vi "Importer.vi"() -> ()   [LabVIEW 2013]
uses:
  Database/Database.lvclass
  <vilib>/addons/database/_DB Variant To Data/Database Variant To Data.xnode
panel:
  in  "mouse tuple":T1={"mouse_id"=1217.0, "mouse_gender"="male", "mouse_strain"="C57BL6/J", "mouse_dob"="", "mouse_dod"="", "mouse_notes"="", "headpost_date"=""}
  out "error":bool
  in  "Import":bool
  in  "stop":bool
  in  "Exo Tuple":T2={"mouse_id"=1217.0, "exp_date"="", "operator"="Manolis", "mass"=0.0, "anesthesia"="fentanyl", "directory"="", "dyes"="OGB", "exp_notes"="", "setup"="2P1", "archive"="", "process"="yes"}
  in  "Tab Control":enum32{"Mouse/Experiment", "Scans"}(tab)
  in  "Archive":string="2PS1A4"
  in  "dyes":string(combo)="OGB"
  in  "Directory":string
  in  "Anesthesia":string(combo)="fentanyl"
  in  "Weight":dbl
  in  "Gender":string(combo)="male"
  in  "Strain":string(combo)="C57BL6/J"
  in  "Birthday":string
  in  "ID":dbl
  in  "Session":path=path "Z:/users/Manolis/Labview/Scanner/sessions_Win7.dsn"
  in  "Mag":dbl=1.0
  in  "Rot":dbl
  in  "Aim":string(combo)="vesselMap"
  in  "Idx":dbl=1.0
  in  "cell #":dbl
  in  "Notes":string
  in  "State":string(combo)="anesthetized"
  in  "File Name":string="vessels"
  in  "Scan Prog":string(combo)="Imager"
  in  "Surface":dbl
  in  "Stim":string(combo)="None"
  in  "Scans":string[][](table)
  in  "Tuple":T3={"mouse_id"=1217.0, "exp_date"="2013-05-16", "scan_idx"=33.0, "file_name"="test", "scan_prog"="Imager", "aim"="other", "stim_engine"="None", "Lens"=0.0, "mag"=0.0, "laser_wavelength"=0.0, "attenuator_setting"=0.0, "x"=0.0, "y"=0.0, "z"=0.0, "surfz"=0.0, "scan_rotation"=0.0, "notes"="", "cell_patch"=0.0, "state"="", "problem_type"=""}
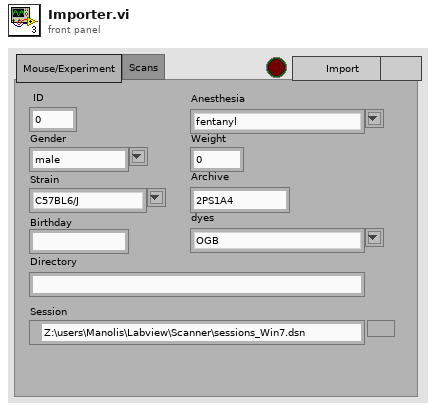
[diagram p1: front panel]
types:
  T1 = cluster{"mouse_id":dbl, "mouse_gender":string, "mouse_strain":string, "mouse_dob":string, "mouse_dod":string, "mouse_notes":string, "headpost_date":string}
  T2 = cluster{"mouse_id":dbl, "exp_date":string, "operator":string, "mass":dbl, "anesthesia":string, "directory":string, "dyes":string, "exp_notes":string, "setup":string, "archive":string, "process":string}
  T3 = cluster{"mouse_id":dbl, "exp_date":string, "scan_idx":dbl, "file_name":string, "scan_prog":string, "aim":string, "stim_engine":string, "Lens":dbl, "mag":dbl, "laser_wavelength":dbl, "attenuator_setting":dbl, "x":dbl, "y":dbl, "z":dbl, "surfz":dbl, "scan_rotation":dbl, "notes":string, "cell_patch":dbl, "state":string, "problem_type":string}
  T4 = cluster{"scan_idx":string, "lens":string, "mag":string, "x":string, "y":string, "z":string, "scan_rotation":string, "scan_prog":string}[]
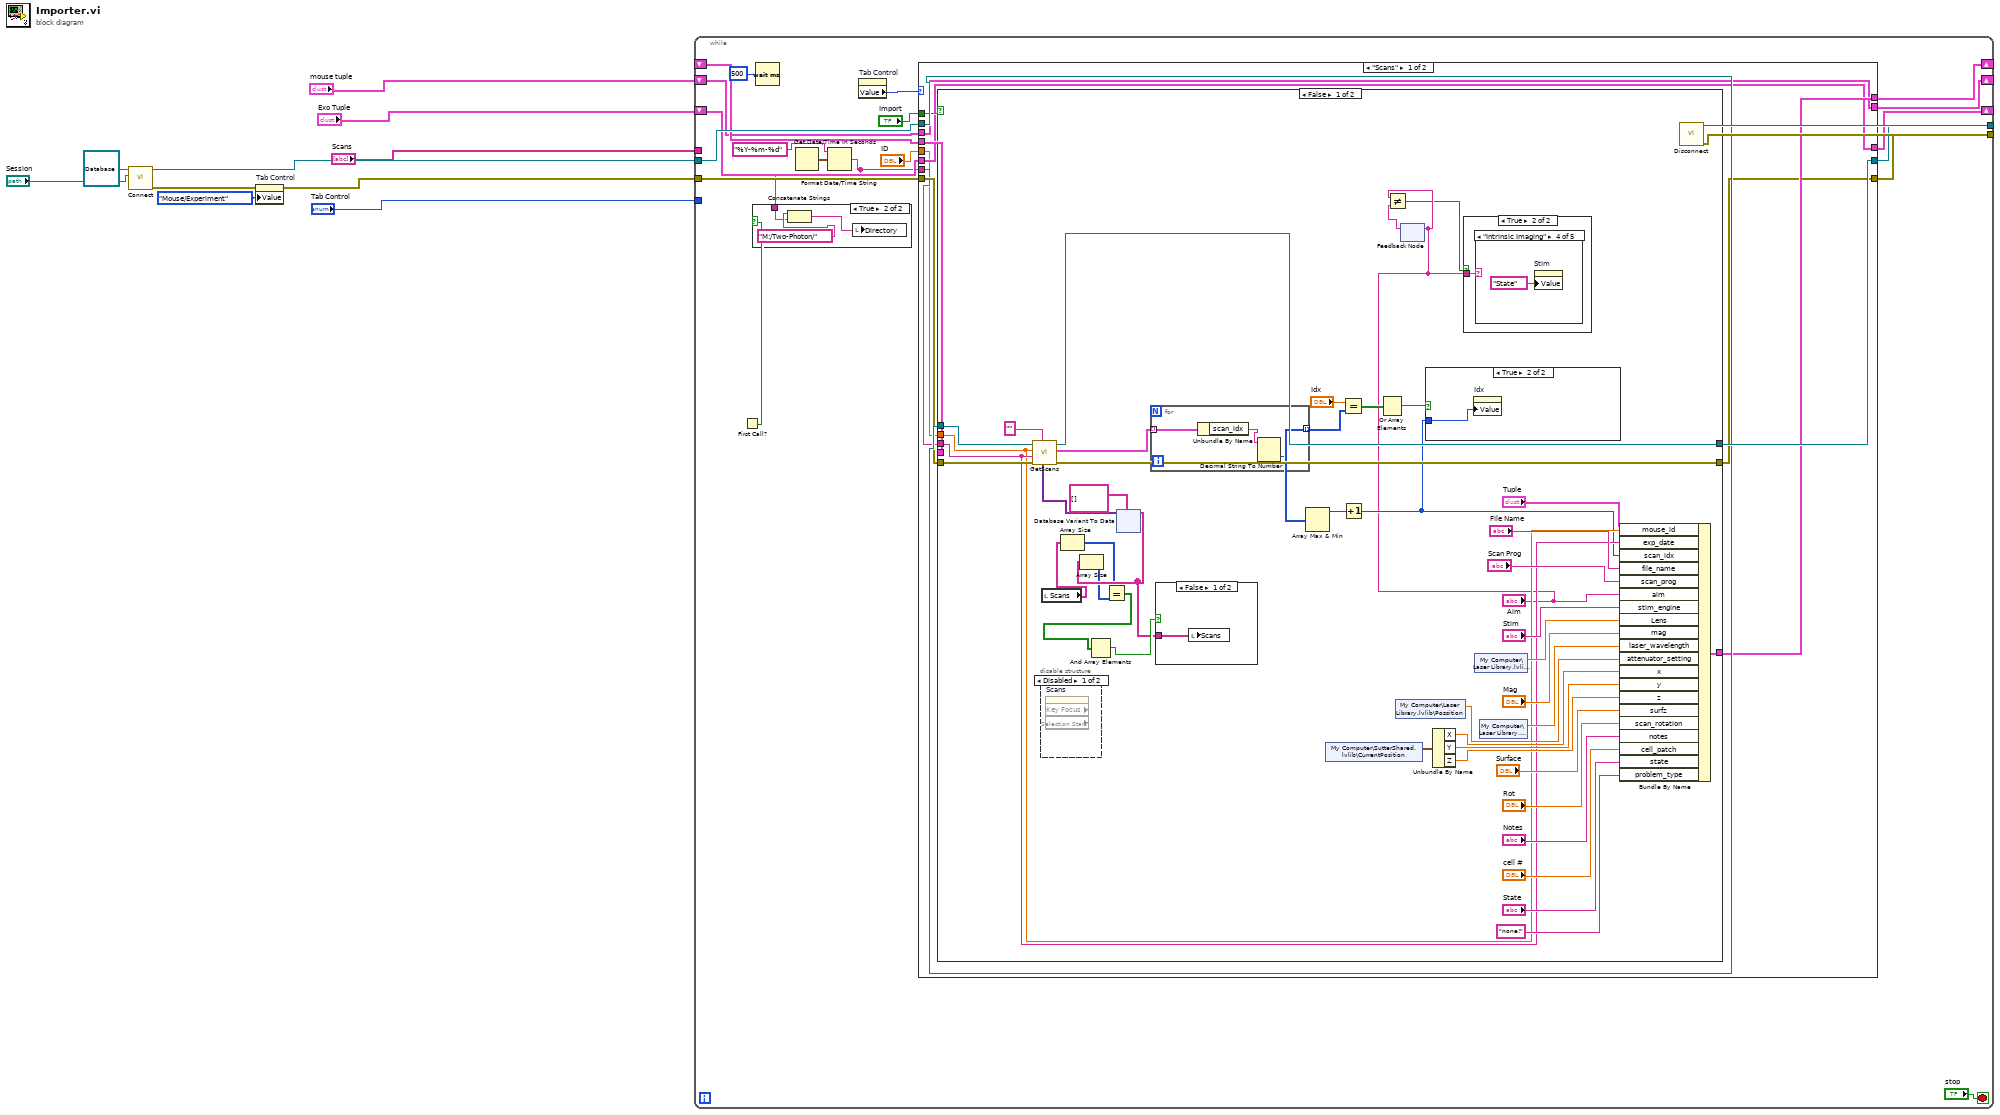
[diagram p0: block diagram]
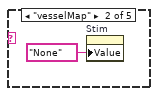
[diagram p5: hidden frame]
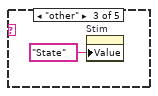
[diagram p6: hidden frame]
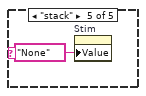
[diagram p7: hidden frame]
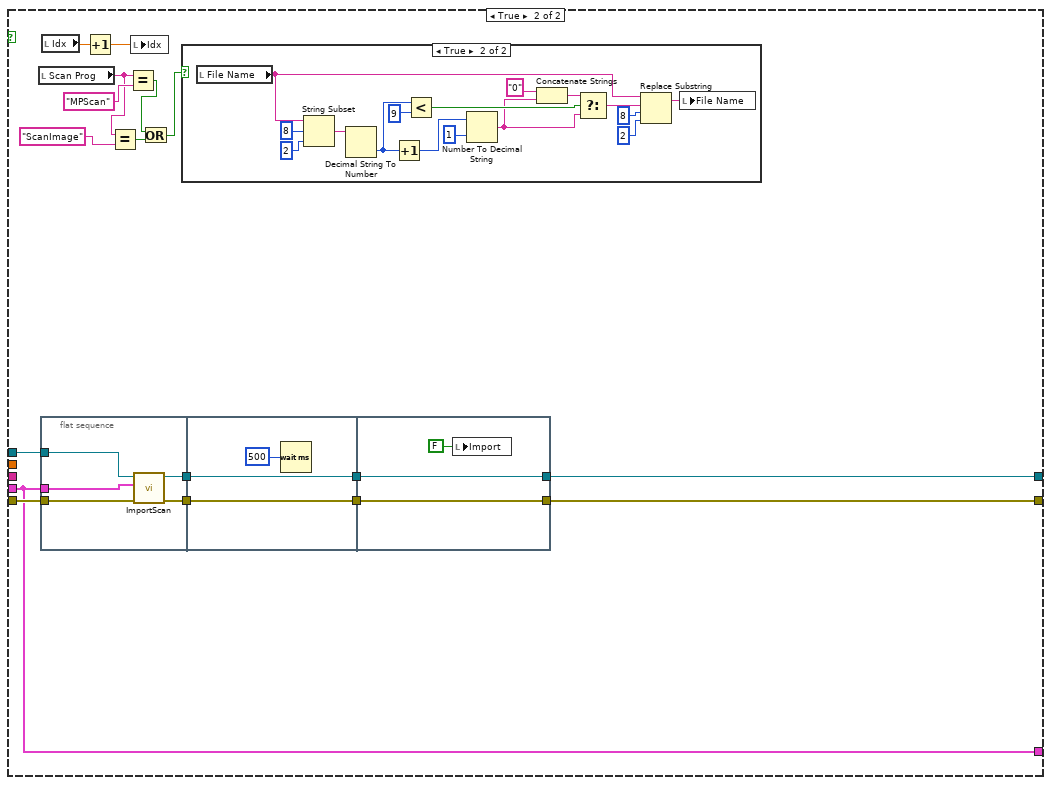
[diagram p11: hidden frame]
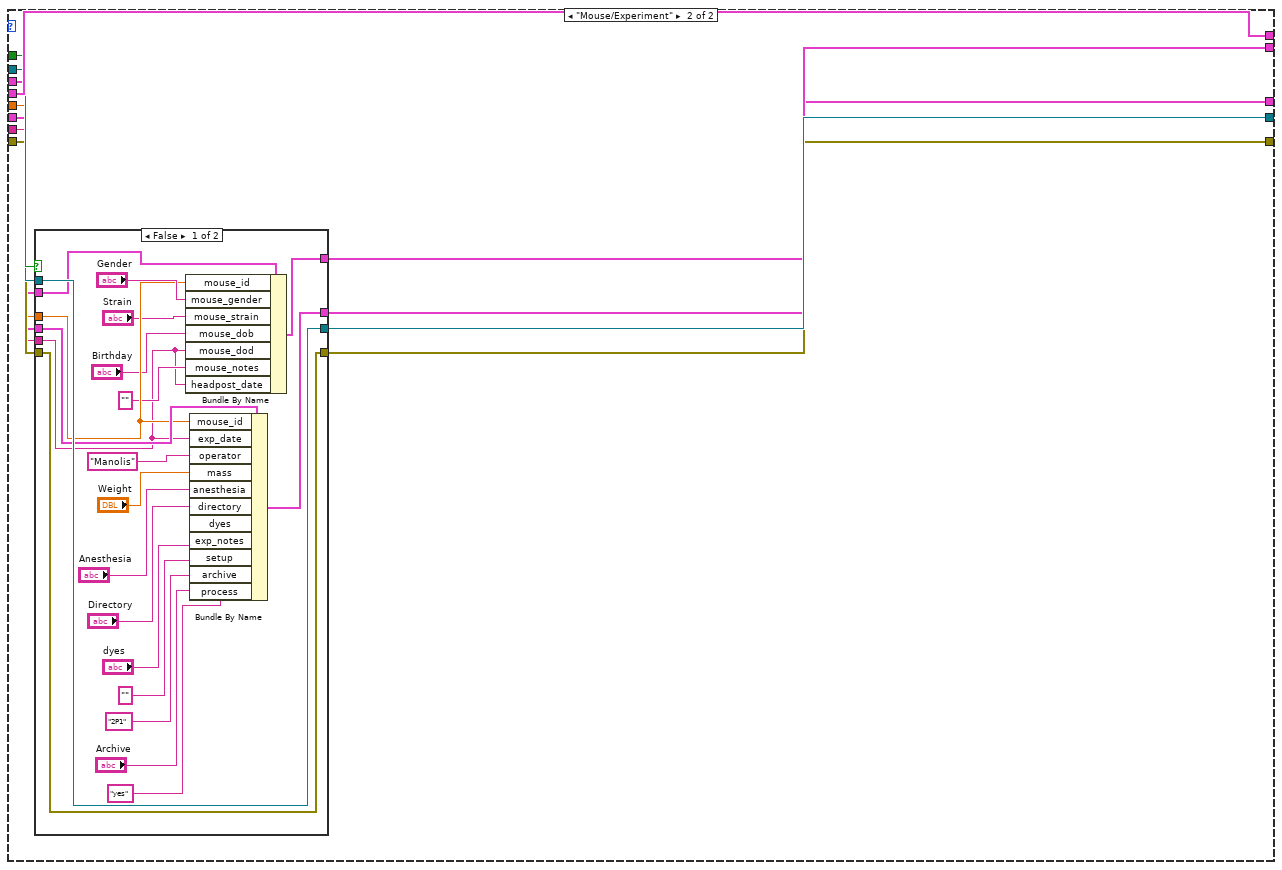
[diagram p13: hidden frame]
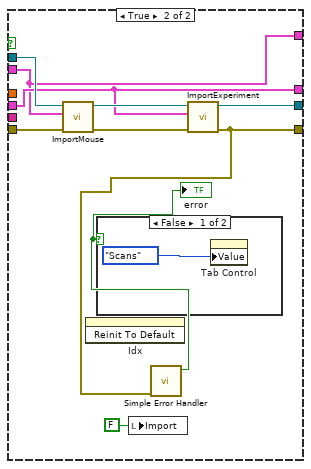
[diagram p14: hidden frame]
diagram:
  n1 = call-dynamic "Connect.vi"("Session"="Session", "Database in"=refnum<class "Database.lvclass"> refnum) -> ("error out"=w4:errorcluster, "Database out"=w10:refnum<class "Database.lvclass">)  [unwired: 8 in]
  n2 = property on="Tab Control" class="TabCtl (strict)"(error in=w4, "Value"=enum32{"Mouse/Experiment", "Scans"}."Mouse/Experiment" ("Tab Control")) -> (error out=w3:errorcluster)  [unwired: 1 in, 1 out]
  n3 = while {
    tunnel: [w31] -> w11
    tunnel: w10 -> [w30]
    tunnel: w3 -> [w28]
    tunnel: [w25] -> w8
    shift-right: [w26] -> _
    shift-left: _ -> [w27]
    tunnel: "Scans" -> [_]
    tunnel: "Tab Control" -> [_]
    shift-right: [w20] -> _
    shift-left: "mouse tuple" -> [w21]
    shift-right: [w18] -> _
    shift-left: "Exo Tuple" -> [w19]
    stop <- "stop" stop-if-true
    n4 = First Call?() -> (First Call?: T/F=w14:bool)
    n5 = Wait (ms)(milliseconds to wait=u32 500) -> ()  [unwired: 1 out]
    n6 = Get Date/Time In Seconds() -> (seconds since 1Jan1904=w23:timestamp)
    n7 = Format Date/Time String(time format string (%c)="%Y-%m-%d", seconds (now)=w23) -> (date/time string=w13:string)  [unwired: 1 in]
    n8 = case shown="True" w14 {
      tunnel: w13 -> [_ w32]
      frame False {
      }
      frame True {
        n9 = Concatenate Strings("M:/Two-Photon/" ("Directory"), w32) -> (w33:string)
        n10 = local write "Directory"(w33) -> ()
      }
    }
    n11 = property on="Tab Control" class="TabCtl (strict)"() -> ("Value"=w16:enum32{"Mouse/Experiment", "Scans"})  [unwired: 2 in, 2 out]
    n12 = case shown="\"Scans\"" w16 {
      tunnel: [w45 w196] -> w31
      tunnel: w30 -> [w44 w197]
      tunnel: w28 -> [w43 w194]
      tunnel: w27 -> [w42 w199]
      tunnel: [w41 w199] -> w26
      tunnel: [w40 w195] -> w25
      tunnel: w13 -> [w39 w188]
      tunnel: "Import" -> [w38 w198]
      tunnel: w21 -> [w37 w193]
      tunnel: [w37 w192] -> w20
      tunnel: w19 -> [w36 w191]
      tunnel: [w36 w190] -> w18
      tunnel: "ID" -> [w35 w189]
      frame "Scans" {
        n13 = case shown="False" w38 {
          tunnel: [w69 w160] -> w45
          tunnel: w44 -> [w70 w159]
          tunnel: w43 -> [w67 w158]
          tunnel: [w66 w157] -> w40
          tunnel: w42 -> [_ w156]
          tunnel: [w72 w156] -> w41
          tunnel: w39 -> [w65 _]
          tunnel: w35 -> [w64 _]
          frame False {
            n14 = call-dynamic "GetScans.vi"("condition"="", "error in (no error)"=w67, "exp_date"=w65, "mouse_id"=w64, "Database in"=w70) -> ("error out"=w66:errorcluster, "Scan Clusters"=w62:T4, "Database out"=w69:refnum<class "Database.lvclass">, "data"=w63:variant[][])  [unwired: 2 in]
            n15 = disable-structure shown="Disabled" {
              frame Disabled {
                n16 = property on="Scans" class="Tbl (strict)" props=["Key Focus", "Selection Start"]() -> ()  [unwired: 2 in, 4 out]
              }
              frame Enabled {
              }
            }
            n17 = local read "Scans"() -> (w51:string[][])
            n18 = Array Size(array=w51) -> (size(s)=w49:i32[])
            n19 = xnode "Database Variant To Data"("database variant"=w63, "type"=string[][] []) -> ("data"=w52:string[][])  [unwired: 1 in, 1 out]
            n20 = Array Size(array=w52) -> (size(s)=w50:i32[])
            n21 = Equal?(x=w49, y=w50) -> (x = y?=w53:bool[])
            n22 = And Array Elements(Boolean array=w53) -> (logical AND=w54:bool)
            n23 = for {
              tunnel: w62 -> [w99] mode=indexing
              tunnel: [w97] -> w60 mode=indexing
              n24 = Unbundle By Name(w99) -> ("scan_idx"=w98:string)
              n25 = Decimal String To Number(string=w98) -> (number=w97:i32)  [unwired: 2 in, 1 out]
            }
            n26 = case shown="False" w54 {
              tunnel: w52 -> [w95 _]
              frame False {
                n27 = local write "Scans"(w95) -> ()
              }
              frame True {
              }
            }
            n28 = Array Max & Min(array=w60) -> (max value=w61:i32)  [unwired: 3 out]
            n29 = shared-variable "My Computer\\SutterShared.lvlib\\CurrentPosition"() -> (w89:cluster{"X":dbl, "Y":dbl, "Z":dbl, "Depth":dbl})  [unwired: 1 in, 1 out]
            n30 = Equal?(x="Idx", y=w60) -> (x = y?=w58:bool[])
            n31 = Increment(x=w61) -> (x+1=w56:i32)
            n32 = Or Array Elements(Boolean array=w58) -> (logical OR=w57:bool)
            n33 = shared-variable "My Computer\\Laser Library.lvlib\\Possition"() -> (w78:dbl)  [unwired: 1 in, 1 out]
            n34 = feedback-in #1("Aim") -> ()
            n35 = feedback #1() -> (w48:string)  [unwired: 1 in]
            n36 = Not Equal?(x="Aim", y=w48) -> (x != y?=w46:bool)
            n37 = case shown="True" w57 {
              tunnel: w56 -> [_ w96]
              frame False {
              }
              frame True {
                n38 = property on="Idx" class="DigNum (strict)"("Value"=w96) -> ()  [unwired: 2 in, 2 out]
              }
            }
            n39 = Unbundle By Name(w89) -> ("X"=w81:dbl, "Y"=w80:dbl, "Z"=w79:dbl)
            n40 = case shown="True" w46 {
              tunnel: "Aim" -> [_ w90]
              frame False {
              }
              frame True {
                n41 = case shown="\"Intrinsic Imaging\"" w90 {
                  frame "False", Default {
                  }
                  frame "vesselMap" {
                    n42 = property on="Stim" class="CmbBox"("Value"="None" ("Stim")) -> ()  [unwired: 2 in, 2 out]
                  }
                  frame "other" {
                    n43 = property on="Stim" class="CmbBox"("Value"="State" ("Stim")) -> ()  [unwired: 2 in, 2 out]
                  }
                  frame "Intrinsic Imaging" {
                    n44 = property on="Stim" class="CmbBox"("Value"="State" ("Stim")) -> ()  [unwired: 2 in, 2 out]
                  }
                  frame "stack" {
                    n45 = property on="Stim" class="CmbBox"("Value"="None" ("Stim")) -> ()  [unwired: 2 in, 2 out]
                  }
                }
              }
            }
            n46 = shared-variable "My Computer\\Laser Library.lvlib\\Lens"() -> (w76:dbl)  [unwired: 1 in, 1 out]
            n47 = shared-variable "My Computer\\Laser Library.lvlib\\WV"() -> (w77:dbl)  [unwired: 1 in, 1 out]
            n48 = Bundle By Name(cluster="Tuple", "mouse_id"=w64, "exp_date"=w65, "scan_idx"=w56, "file_name"="File Name", "scan_prog"="Scan Prog", "aim"="Aim", "stim_engine"="Stim", "Lens"=w76, "mag"="Mag", "laser_wavelength"=w77, "attenuator_setting"=w78, "x"=w81, "y"=w80, "z"=w79, "surfz"="Surface", "scan_rotation"="Rot", "notes"="Notes", "cell_patch"="cell #", "state"="State", "problem_type"="none!") -> (w72:T3)
          }
          frame True {
            n49 = local read "Scan Prog"() -> (w145:string)
            n50 = flat-sequence {
              tunnel: w159 -> [w164]
              tunnel: w158 -> [w163]
              tunnel: w156 -> [w161]
              tunnel: [w165] -> w152
              tunnel: [w162] -> w151
              tunnel: w152 -> [w168]
              tunnel: w151 -> [w167]
              tunnel: [w168] -> w150
              tunnel: [w167] -> w149
              tunnel: [w170] -> w157
              tunnel: [w171] -> w160
              tunnel: w150 -> [w171]
              tunnel: w149 -> [w170]
              frame #0 {
                n51 = call-dynamic "ImportScan.vi"("error in (no error)"=w163, "Tuple"=w161, "Database in"=w164) -> ("error out"=w162:errorcluster, "Database out"=w165:refnum<class "Database.lvclass">)  [unwired: 7 in]
              }
              frame #1 {
                n52 = Wait (ms)(milliseconds to wait=u32 500) -> ()  [unwired: 1 out]
              }
              frame #2 {
                n53 = local write "Import"(FALSE ("Import")) -> ()
              }
            }
            n54 = local read "Idx"() -> (w155:dbl)
            n55 = Increment(x=w155) -> (x+1=w154:dbl)
            n56 = Equal?(x=w145, y="ScanImage") -> (x = y?=w148:bool)
            n57 = Equal?(x=w145, y="MPScan") -> (x = y?=w147:bool)
            n58 = local write "Idx"(w154) -> ()
            n59 = Or(x=w147, y=w148) -> (x .or. y?=w146:bool)
            n60 = case shown="True" w146 {
              frame False {
              }
              frame True {
                n61 = local read "File Name"() -> (w173:string)
                n62 = String Subset(string=w173, offset (0)=8, length (rest)=2 ("length (rest)")) -> (substring=w185:string)
                n63 = Decimal String To Number(string=w185) -> (number=w179:i32)  [unwired: 2 in, 1 out]
                n64 = Increment(x=w179) -> (x+1=w184:i32)
                n65 = Less?(x=w179, y=9) -> (x < y?=w178:bool)
                n66 = Number To Decimal String(number=w184, width (-)=i16 1) -> (decimal integer string=w175:string)
                n67 = Concatenate Strings("0", w175) -> (w176:string)
                n68 = Select(t=w176, s=w178, f=w175) -> (s? t:f=w174:string)
                n69 = Replace Substring(2:2 ("length (len. of substring)"), 3:8 ("offset (0)"), 4:w174, 5:w173) -> (1:w172:string)  [unwired: 1 out]
                n70 = local write "File Name"(w172) -> ()
              }
            }
          }
        }
      }
      frame "Mouse/Experiment" {
        n71 = case shown="False" w198 {
          tunnel: w197 -> [w220 w230]
          tunnel: [w220 w226] -> w196
          tunnel: [w219 w223] -> w195
          tunnel: w194 -> [w219 w229]
          tunnel: w193 -> [w207 w224]
          tunnel: [w201 w224] -> w192
          tunnel: w191 -> [w218 w225]
          tunnel: [w217 w225] -> w190
          tunnel: w189 -> [w205 _]
          tunnel: w188 -> [w200 _]
          frame False {
            n72 = Bundle By Name(cluster=w207, "mouse_id"=w205, "mouse_gender"="Gender", "mouse_strain"="Strain", "mouse_dob"="Birthday", "mouse_dod"=w200, "mouse_notes"="", "headpost_date"=w200) -> (w201:T1)
            n73 = Bundle By Name(cluster=w218, "mouse_id"=w205, "exp_date"=w200, "operator"="Manolis", "mass"="Weight", "anesthesia"="Anesthesia", "directory"="Directory", "dyes"="dyes", "exp_notes"="", "setup"="2P1", "archive"="Archive", "process"="yes") -> (w217:T2)
          }
          frame True {
            n74 = call-dynamic "ImportMouse.vi"("error in (no error)"=w229, "Tuple"=w224, "Database in"=w230) -> ("error out"=w228:errorcluster, "Database out"=w227:refnum<class "Database.lvclass">)  [unwired: 7 in]
            n75 = invoke on="Idx" class="DigNum (strict)" method="Reinit To Default"() -> ()  [unwired: 3 in, 3 out]
            n76 = local write "Import"(FALSE ("Import")) -> ()
            n77 = call-dynamic "ImportExperiment.vi"("error in (no error)"=w228, "Tuple"=w225, "Database in"=w227) -> ("error out"=w223:errorcluster, "Database out"=w226:refnum<class "Database.lvclass">)  [unwired: 7 in]
            n78 = call <vilib>:"Simple Error Handler.vi"("error in (no error)"=w223) -> ("error?"=w222:bool)  [unwired: 4 in, 4 out]
            "error" <- w222
            n79 = case shown="False" w222 {
              frame False {
                n80 = property on="Tab Control" class="TabCtl (strict)"("Value"=enum32{"Mouse/Experiment", "Scans"}."Scans" ("Tab Control")) -> ()  [unwired: 2 in, 2 out]
              }
              frame True {
              }
            }
          }
        }
      }
    }
  }
  n81 = call-dynamic "Disconnect.vi"("error in (no error)"=w8, "Database in"=w11) -> ()  [unwired: 8 in, 2 out]
